vi "Init.vi"(8 "error in (no error)":errorcluster, 11 "BetterMultiListboxHandle in":refnum<class "BetterMultiListboxHandle.lvclass">) -> (0 "error out":errorcluster, 3 "BetterMultiListboxHandle out":refnum<class "BetterMultiListboxHandle.lvclass">)   [LabVIEW 2020, in "BetterDragAndDrop.lvlib" / "BetterMultiListboxHandle.lvclass"]
uses:
  BetterMultiListboxHandle.lvclass
  C:/DSCE code/Open-source/betterdraganddrop_GIT/Source/Classes/BetterHandle/BetterHandle.lvclass
  BetterMultiListboxHandle.lvclass/BetterMultiListboxHandle.ctl
  <vilib>/Utility/miscctls.llb/LVRowAndColumnTypeDef.ctl
  BetterHandle/Pixel Constants.ctl
  BetterHandle/BetterHandle.lvclass/BetterHandle.ctl
  BetterHandle/Write Constant Sizes.vi
  BetterHandle/BetterHandle.lvclass
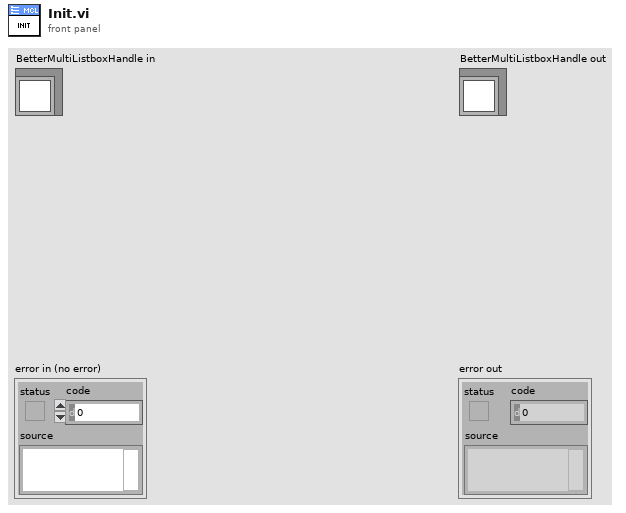
[diagram p1: front panel]
types:
  T1 = typedef "BetterDragAndDrop.lvlib/BetterHandle.lvclass/Pixel Constants.ctl" = cluster{"Row Header height":i32, "Row height":i32, "Column Header Offset":i32}
  T2 = typedef "LVRowAndColumnTypeDef.ctl" = cluster{"Row":i32, "Column":i32}
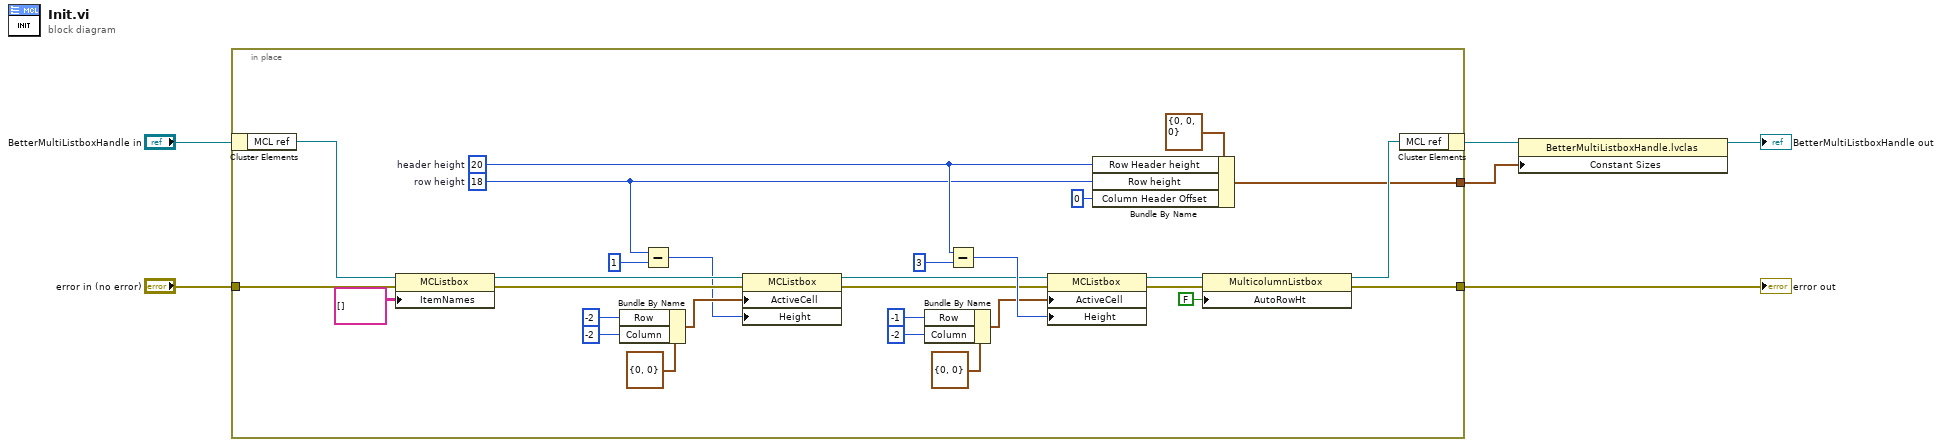
[diagram p0: block diagram]
diagram:
  n1 = in-place {
    in-place-border: "error in (no error)" -> [w34]
    in-place-border: [w13] -> w4
    in-place-border: [w7] -> w1
    w9 = 18  # row height
    w10 = 20  # header height
    n2 = in-place-cluster #1("BetterMultiListboxHandle in") -> ("MCL ref"=w35:refnum<vi>)
    n3 = property class="MCListbox"(reference=w35, error in=w34, "ItemNames"=string[][] [] ("Item Names")) -> (reference out=w28:refnum<vi>, error out=w27:errorcluster)
    n4 = Bundle By Name(cluster=T2 {"Row"=0, "Column"=0} ("Active Cell:Active Cell"), "Row"=-2, "Column"=-2) -> (w29:T2)
    n5 = Subtract(x=w9, y=1) -> (x-y=w25:i32)
    n6 = property class="MCListbox"(reference=w28, error in=w27, "ActiveCell"=w29, "Height"=w25) -> (reference out=w18:refnum<vi>, error out=w17:errorcluster)
    n7 = Bundle By Name(cluster=T2 {"Row"=0, "Column"=0} ("Active Cell:Active Cell"), "Row"=-1, "Column"=-2) -> (w22:T2)
    n8 = Subtract(x=w10, y=3) -> (x-y=w24:i32)
    n9 = property class="MCListbox"(reference=w18, error in=w17, "ActiveCell"=w22, "Height"=w24) -> (reference out=w12:refnum<vi>, error out=w16:errorcluster)
    n10 = Bundle By Name(cluster=T1 {"Row Header height"=0, "Row height"=0, "Column Header Offset"=0} ("Constant Sizes"), "Row Header height"=w10, "Row height"=w9, "Column Header Offset"=0) -> (w7:T1)
    n11 = property class="MulticolumnListbox"(reference=w12, error in=w16, "AutoRowHt"=FALSE ("Autosizing Row Height")) -> (reference out=w14:refnum<vi>, error out=w13:errorcluster)
    n12 = in-place-cluster #1("MCL ref"=w14) -> (w3:refnum<class "BetterMultiListboxHandle.lvclass">)
  }
  "error out" <- w4
  n13 = property class="BetterMultiListboxHandle.lvclas"(reference=w3, "Constant Sizes"=w1) -> (reference out=→"BetterMultiListboxHandle out":refnum<class "BetterMultiListboxHandle.lvclass">)  [unwired: 1 in, 1 out]
